vi "DTbl Uncompress Digital.vi"(8 "error in (no error)":errorcluster, 11 "digital data in":digitaldata) -> (0 "error out":errorcluster, 3 "digital data out":digitaldata)   [LabVIEW 2011]
doc: "Uncompresses the digital signals in the digital input and returns the result in the digital output. Wire data to the <B>uncompressed digital waveform</B> input to determine the polymorphic instance to use or manually select the instance."
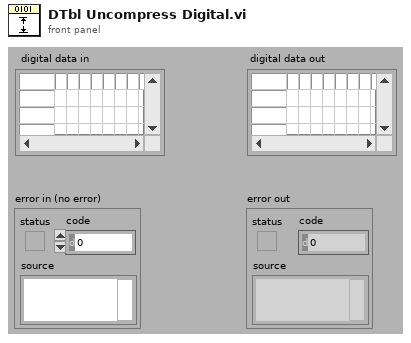
[diagram p1: front panel]
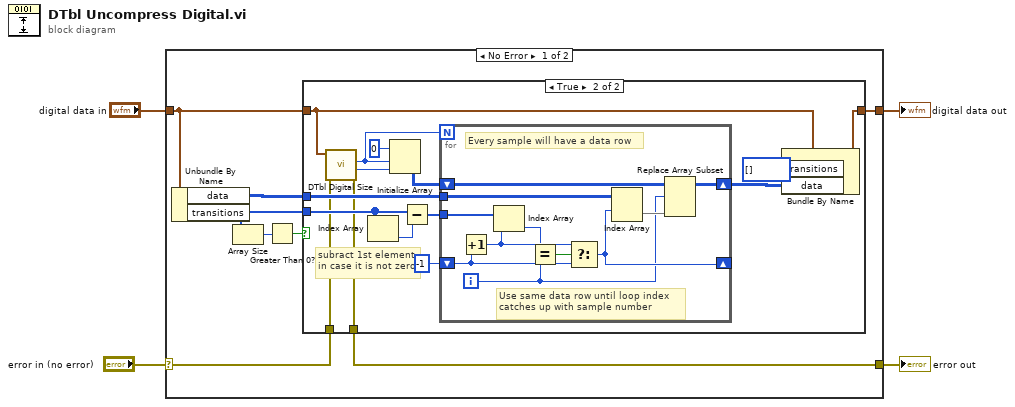
[diagram p0: block diagram]
diagram:
  n1 = case shown="No Error" "error in (no error)" {
    selector: "error in (no error)" -> [w6 w42]
    tunnel: [w12 w41] -> w4
    tunnel: "digital data in" -> [w9 w41]
    tunnel: [w5 w42] -> w1
    frame No Error {
      n2 = Unbundle By Name(w9) -> ("data"=w8:u8[][], "transitions"=w7:u32[])
      n3 = Array Size(array=w7) -> (size(s)=w11:i32)
      n4 = Greater Than 0?(x=w11) -> (x > 0?=w10:bool)
      n5 = case shown="True" w10 {
        tunnel: w8 -> [_ w25]
        tunnel: [w14 w20] -> w12
        tunnel: w9 -> [w14 w15]
        tunnel: w7 -> [_ w18]
        tunnel: w6 -> [w13 w17]
        tunnel: [w13 w16] -> w5
        frame False {
          # "NOT Compressed"
        }
        frame True {
          # "subract 1st element\nin case it is not zero"
          n6 = call "DTbl Digital Size.vi"("error in (no error)"=w17, "digital data in"=w15) -> ("error out"=w16:errorcluster, "number of signals"=w28:i32, "number of samples"=w27:i32)  [unwired: 6 in, 1 out]
          n7 = Index Array(array=w18) -> (element=w23:u32)  [unwired: 1 in]
          n8 = Initialize Array(u8 0, w27, w28) -> (w19:u8[][])
          n9 = Subtract(x=w18, y=w23) -> (x-y=w24:u32[])
          n10 = for {
            N: w27 -> [_]
            shift-right: [w36] -> w21
            shift-left: w19 -> [w37]
            shift-right: [w34] -> _
            shift-left: -1 -> [w30]
            tunnel: w24 -> [w40]
            tunnel: w25 -> [w38]
            i -> [w31]
            # "Use same data row until loop index \ncatches up with sample number"
            # "Every sample will have a data row"
            n11 = Increment(x=w30) -> (x+1=w33:i32)
            n12 = Index Array(array=w40, index=w33) -> (element=w32:u32)
            n13 = Equal?(x=w32, y=w31) -> (x = y?=w39:bool)
            n14 = Select(t=w33, s=w39, f=w30) -> (s? t:f=w34:i32)
            n15 = Index Array(array=w38, index (row)=w34) -> (element=w35:u8[])  [unwired: 1 in]
            n16 = Replace Array Subset(array=w37, new element=w35, index (row)=w31) -> (w36:u8[][])  [unwired: 1 in]
          }
          n17 = Bundle By Name(cluster=w15, "transitions"=u32[] [] ("Samples"), "data"=w21) -> (w20:digitaldata)
        }
      }
    }
    frame Error {
    }
  }
  "digital data out" <- w4
  "error out" <- w1
